vi "Sensors.vi"() -> ()   [LabVIEW 2018]
uses:
  <vilib>/Rock Robotics/SystemInterfaces/DIO/FPGA_DIOChannel.ctl
  <vilib>/Rock Robotics/WPI/Switch/WPI_SwitchOpenLimit.vi
  Sensors Global.vi
  Times/Times Global.vi
panel:
  in  "Stop VI":bool
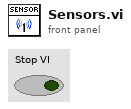
[diagram p1: front panel]
types:
  T1 = typedef "FPGA_DIOChannel.ctl" = enum8{"DIO 0", "DIO 1", "DIO 2", "DIO 3", "DIO 4", "DIO 5", "DIO 6", "DIO 7", "DIO 8", "DIO 9", "DIO MXP 0", "DIO MXP 1", "DIO MXP 2", "DIO MXP 3", "DIO MXP 4", "DIO MXP 5", "DIO MXP 6", "DIO MXP 7", "DIO MXP 8", "DIO MXP 9", "DIO MXP 10", "DIO MXP 11", "DIO MXP 12", "DIO MXP 13", "DIO MXP 14", "DIO MXP 15", "SPI Port CS1", "SPI Port CS2", "SPI Port CS3", "SPI Port MISO", "SPI Port MOSI", "Invalid"}
  T2 = typedef "WPI_SwitchDevRef.ctl" = cluster{"DevStatus":errorcluster, "DIO Channel":T1, "CntIndex":T3, "Normally Closed":bool}
  T3 = typedef "FPGA_CounterCtrSystemIndex.ctl" = enum8{"Ctr 0", "Ctr 1", "Ctr 2", "Ctr 3", "Ctr 4", "Ctr 5", "Ctr 6", "Ctr 7", "Invalid"}
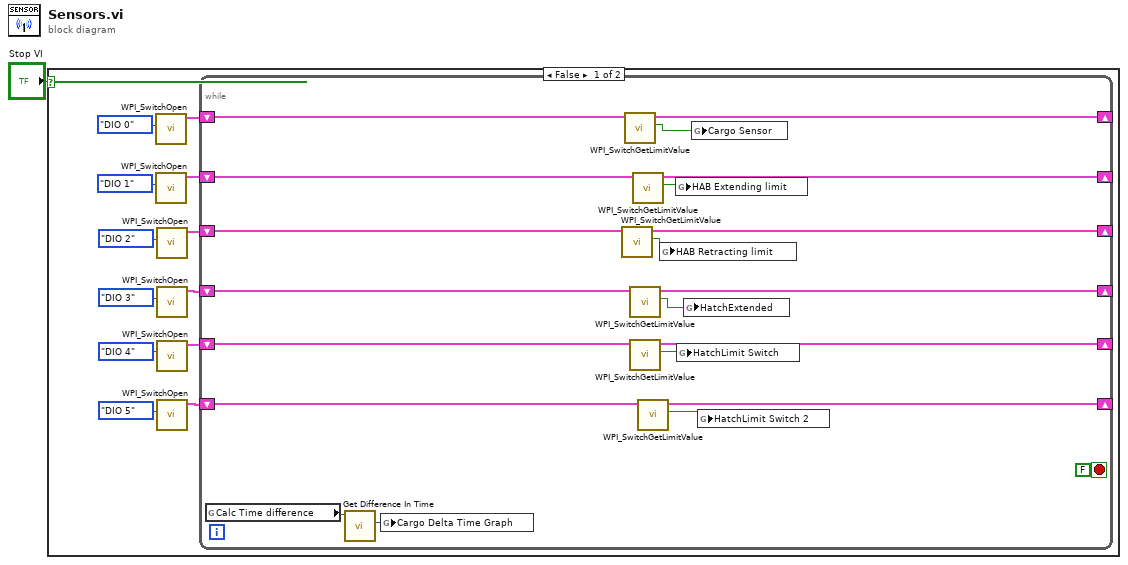
[diagram p0: block diagram]
diagram:
  n1 = case shown="False" "Stop VI" {
    frame False {
      n2 = call-poly <vilib>:"WPI_SwitchOpen.vi"("DIO Channel"=FPGA_DIOChannel."DIO 0") -> ("SwitchDevRef"=w12:T2)  [unwired: 9 in, 1 out]
      n3 = call-poly <vilib>:"WPI_SwitchOpen.vi"("DIO Channel"=FPGA_DIOChannel."DIO 1") -> ("SwitchDevRef"=w7:T2)  [unwired: 9 in, 1 out]
      n4 = call-poly <vilib>:"WPI_SwitchOpen.vi"("DIO Channel"=FPGA_DIOChannel."DIO 2") -> ("SwitchDevRef"=w6:T2)  [unwired: 9 in, 1 out]
      n5 = call-poly <vilib>:"WPI_SwitchOpen.vi"("DIO Channel"=FPGA_DIOChannel."DIO 3") -> ("SwitchDevRef"=w5:T2)  [unwired: 9 in, 1 out]
      n6 = call-poly <vilib>:"WPI_SwitchOpen.vi"("DIO Channel"=FPGA_DIOChannel."DIO 4") -> ("SwitchDevRef"=w4:T2)  [unwired: 9 in, 1 out]
      n7 = call-poly <vilib>:"WPI_SwitchOpen.vi"("DIO Channel"=FPGA_DIOChannel."DIO 5") -> ("SwitchDevRef"=w3:T2)  [unwired: 9 in, 1 out]
      n8 = while {
        shift-right: [w30] -> _
        shift-left: w12 -> [w31]
        shift-right: [w29] -> _
        shift-left: w7 -> [w28]
        shift-right: [w26] -> _
        shift-left: w6 -> [w23]
        shift-right: [w27] -> _
        shift-left: w5 -> [w22]
        shift-right: [w25] -> _
        shift-left: w4 -> [w21]
        shift-right: [w24] -> _
        shift-left: w3 -> [w20]
        stop <- FALSE stop-if-true
        n9 = global read "Sensors Global.vi" "Calc Time difference"() -> (w33:bool)
        n10 = call "Get Difference In Time.vi"("Calculate Time Difference"=w33) -> ("Delta Time over Time"=w32:u32)  [unwired: 9 in, 1 out]
        n11 = global write "Times Global.vi" "Cargo Delta Time Graph"(w32) -> ()
        n12 = call <vilib>:"WPI_SwitchGetLimitValue.vi"("SwitchDevRef"=w23) -> ("Switch Pressed"=w16:bool, "SwitchDevRef"=w26:T2)  [unwired: 8 in, 1 out]
        n13 = call <vilib>:"WPI_SwitchGetLimitValue.vi"("SwitchDevRef"=w31) -> ("Switch Pressed"=w19:bool, "SwitchDevRef"=w30:T2)  [unwired: 8 in, 1 out]
        n14 = call <vilib>:"WPI_SwitchGetLimitValue.vi"("SwitchDevRef"=w22) -> ("Switch Pressed"=w15:bool, "SwitchDevRef"=w27:T2)  [unwired: 8 in, 1 out]
        n15 = call <vilib>:"WPI_SwitchGetLimitValue.vi"("SwitchDevRef"=w21) -> ("Switch Pressed"=w14:bool, "SwitchDevRef"=w25:T2)  [unwired: 8 in, 1 out]
        n16 = call <vilib>:"WPI_SwitchGetLimitValue.vi"("SwitchDevRef"=w28) -> ("Switch Pressed"=w17:bool, "SwitchDevRef"=w29:T2)  [unwired: 8 in, 1 out]
        n17 = call <vilib>:"WPI_SwitchGetLimitValue.vi"("SwitchDevRef"=w20) -> ("Switch Pressed"=w18:bool, "SwitchDevRef"=w24:T2)  [unwired: 8 in, 1 out]
        n18 = global write "Sensors Global.vi" "HAB Retracting limit"(w16) -> ()
        n19 = global write "Sensors Global.vi" "HAB Extending limit"(w17) -> ()
        n20 = global write "Sensors Global.vi" "HatchLimit Switch"(w14) -> ()
        n21 = global write "Sensors Global.vi" "HatchExtended"(w15) -> ()
        n22 = global write "Sensors Global.vi" "Cargo Sensor"(w19) -> ()
        n23 = global write "Sensors Global.vi" "HatchLimit Switch 2"(w18) -> ()
      }
    }
    frame True {
    }
  }
